vi "Get_Temperature.vi"(5 "Close visa session":bool=TRUE, 7 "Res?":bool, 9 "Controller":u16(ring) items=["LS370", "LS340", "LS336"], 10 "Channel":u16(ring) items=["A", "B", "C", "D", "4"], 11 "VISA resource name":refnum<visa-resource-name>) -> (3 "Temperature":dbl)   [LabVIEW 2019]
panel:
  in  "error in (no error)":errorcluster
  out "error out":errorcluster
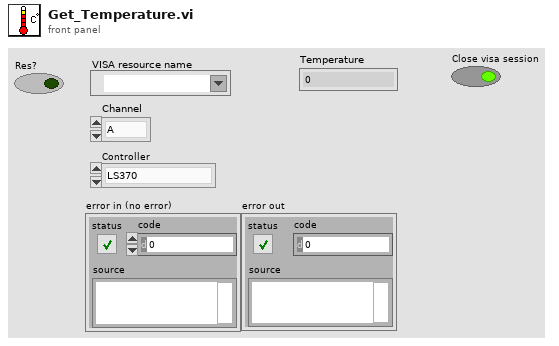
[diagram p1: front panel]
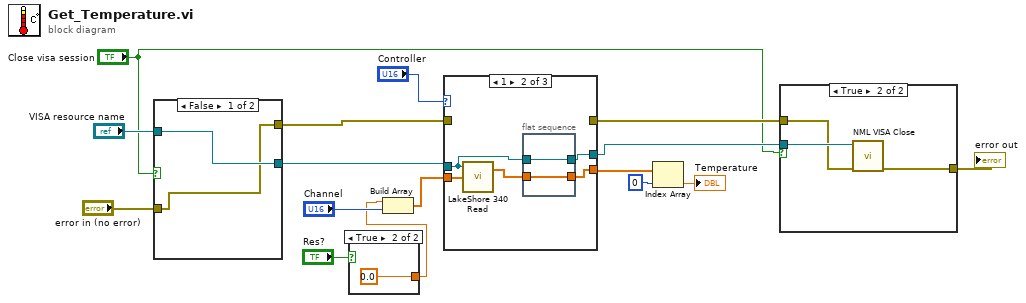
[diagram p0: block diagram]
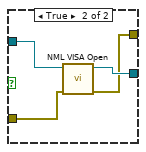
[diagram p3: hidden frame]
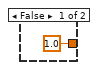
[diagram p4: hidden frame]
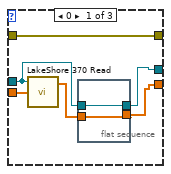
[diagram p5: hidden frame]
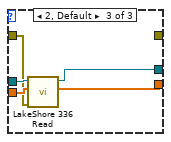
[diagram p6: hidden frame]
diagram:
  n1 = case shown="False" "Close visa session" {
    tunnel: "VISA resource name" -> [w18 w22]
    tunnel: [w18 w21] -> w7
    tunnel: [w17 w20] -> w6
    tunnel: "error in (no error)" -> [w17 w19]
    frame False {
    }
    frame True {
      n2 = call "NML VISA Open.vi"("error in (no error)"=w19, "VISA resource name"=w22) -> ("error out"=w20:errorcluster, "VISA resource name out"=w21:refnum<visa-resource-name>)  [unwired: 8 in]
    }
  }
  n3 = case shown="True" "Res?" {
    tunnel: [1.0 ("element") 0.0 ("element")] -> w9
    frame False {
    }
    frame True {
    }
  }
  n4 = Build Array(w9, "Channel") -> (w13:dbl[])
  n5 = case shown="1" "Controller" {
    tunnel: w7 -> [w26 w36 w44]
    tunnel: w6 -> [w29 _ w40]
    tunnel: [w27 w34 w42] -> w16
    tunnel: w13 -> [w30 w37 w43]
    tunnel: [w29 _ _] -> w3
    tunnel: [w25 w35 w41] -> w5
    frame 0 {
      n6 = call "LakeShore 370 Read.vi"("Parameters"=w30, "Instrument Address"=w26) -> ("Measurement"=w28:dbl[])  [unwired: 1 in, 1 out]
      n7 = flat-sequence {
        tunnel: w28 -> [w32]
        tunnel: [w32] -> w27
        tunnel: w26 -> [w31]
        tunnel: [w31] -> w25
        frame #0 {
        }
      }
    }
    frame 1 {
      n8 = call "LakeShore 340 Read.vi"("Parameters"=w37, "Instrument Address"=w36) -> ("Measurement"=w33:dbl[])  [unwired: 1 in, 1 out]
      n9 = flat-sequence {
        tunnel: w36 -> [w39]
        tunnel: [w39] -> w35
        tunnel: [w38] -> w34
        tunnel: w33 -> [w38]
        frame #0 {
        }
      }
    }
    frame 2, Default {
      n10 = call "LakeShore 336 Read.vi"("error in (no error)"=w40, "Parameters"=w43, "Instrument Address"=w44) -> ("Measurement"=w42:dbl[], "dup VISA session"=w41:refnum<visa-resource-name>)  [unwired: 1 in, 2 out]
    }
  }
  n11 = Index Array(array=w16, index=0) -> (element=→"Temperature":dbl)
  n12 = case shown="True" "Close visa session" {
    tunnel: w5 -> [_ w48]
    tunnel: [w45 w47] -> w4
    tunnel: w3 -> [w45 w46]
    frame False {
    }
    frame True {
      n13 = call "NML VISA Close.vi"("Error In"=w46, "VISA resource name"=w48) -> ("Error Out"=w47:errorcluster)  [unwired: 9 in]
    }
  }
  "error out" <- w4
